vi "I32 Value.vi"(8 "error in (no error)":errorcluster, 11 "Double Float in":refnum<class "Complex Single Float.lvclass">) -> (0 "error out":errorcluster, 2 "I32":i32, 3 "Double Float out":refnum<class "Complex Single Float.lvclass">)   [LabVIEW 2021, in "Complex Single Float.lvclass"]
uses:
  Complex Single Float.lvclass
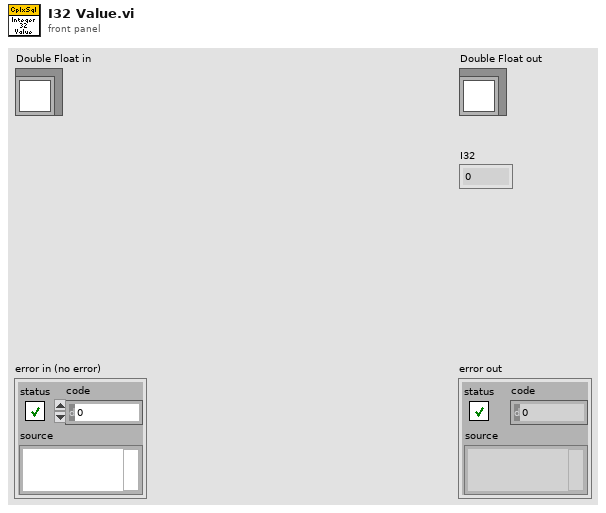
[diagram p1: front panel]
types:
  T1 = typedef "Complex Single Float.lvclass/Type.ctl" = csg
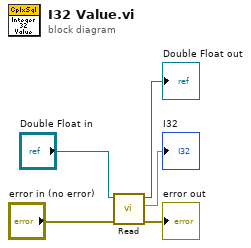
[diagram p0: block diagram]
diagram:
  n1 = call-dynamic "Read.vi"("error in (no error)"="error in (no error)", "Double Float.lvclass_340760 in"="Double Float in") -> ("error out"=→"error out":errorcluster, "Value"=→"I32":T1, "Double Float.lvclass_340760 out"=→"Double Float out":refnum<class "Complex Single Float.lvclass">)  [unwired: 7 in]
